vi "ReturnInterfaceReference.vi"(8 "error in (no error)":errorcluster, 11 "CreateInterface in":refnum<class "CreateInterface.lvclass">) -> (0 "error out":errorcluster, 2 "IntRef":refnum<vi>, 3 "CreateInterface out":refnum<class "CreateInterface.lvclass">)   [LabVIEW 2020, in "Mermaid.lvlib" / "CreateInterface.lvclass"]
uses:
  CreateInterface.lvclass
  CreateInterface.lvclass/CreateInterface.ctl
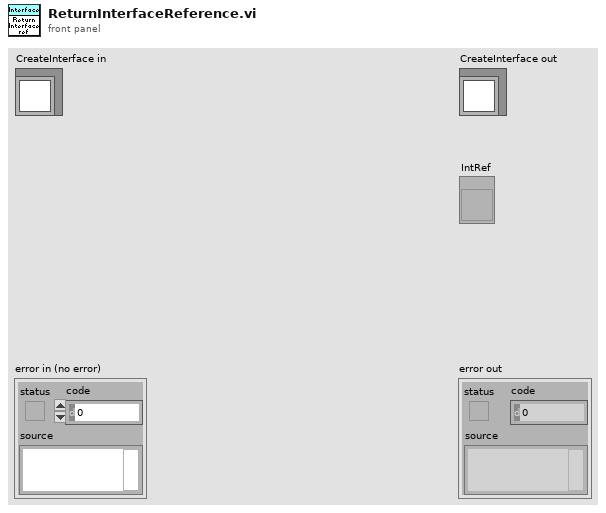
[diagram p1: front panel]
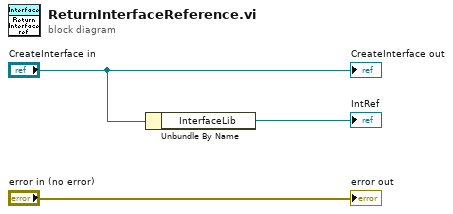
[diagram p0: block diagram]
diagram:
  n1 = Unbundle By Name("CreateInterface in") -> ("InterfaceLib"=→"IntRef":refnum<vi>)
  "error out" <- "error in (no error)"
  "CreateInterface out" <- "CreateInterface in"
